vi "png_to_colors.vi"(11 "colors":string(combo)="parula") -> (3 "colors":u32[](array[colorbox]))   [LabVIEW 2019, in "Mandelbrot.lvlib"]
uses:
  Mandelbrot.lvlib
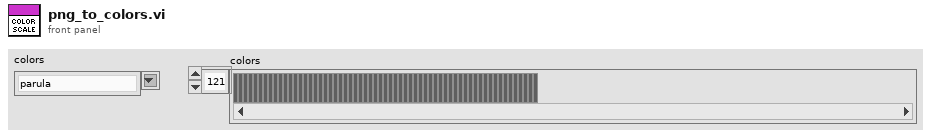
[diagram p1: front panel]
types:
  T1 = typedef "imagedata.ctl" = cluster{"image type":i32, "image depth":i32, "image":u8[], "mask":u8[], "colors":u32[], "Rectangle":cluster{"left":i16, "top":i16, "right":i16, "bottom":i16}}
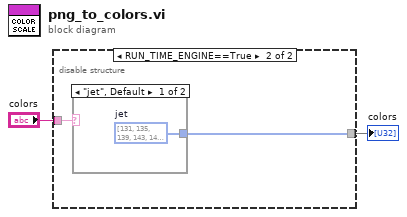
[diagram p0: block diagram]
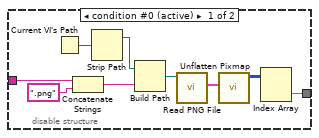
[diagram p2: hidden frame]
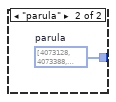
[diagram p3: hidden frame]
diagram:
  n1 = disable-structure shown="RUN_TIME_ENGINE==True" {
    disable-tunnel: [w6 w12] -> w2
    disable-tunnel: "colors" -> [w5 w13]
    frame condition #0 (active) {
      n2 = Current VI's Path() -> (path=w11:path)
      n3 = Concatenate Strings(w5, ".png" ("string")) -> (w3:string)
      n4 = Strip Path(path=w11) -> (stripped path=w10:path)  [unwired: 1 out]
      n5 = Build Path(base path=w10, name or relative path=w3) -> (appended path=w9:path)
      n6 = call <vilib>:"Read PNG File.vi"("path to PNG file"=w9) -> ("image data"=w8:T1)  [unwired: 8 in, 2 out]
      n7 = call <vilib>:"Unflatten Pixmap.vi"("image data"=w8) -> ("24-bit pixmap"=w7:u32[][])  [unwired: 4 in, 6 out]
      n8 = Index Array(array=w7) -> (element=w6:u32[])  [unwired: 2 in]
    }
    frame condition #1 {
      n9 = case shown="\"jet\", Default" w13 {
        tunnel: [w14 w15] -> w12
        frame "jet", Default {
          w14 = u32[] [131, 135, 139, 143, 147, 151, 155, 159, 163, 167, 172, 175, 179, 183, 186, 191, 195, 198, 203, 207, 211, 215, 219, 223, 227, 231, 235, 239, 243, 247, 251, 255, 1279, 2303, 3327, 4607, 5375, 6399, 7423, 8191, 9471, 10495, 11263, 12543, 13567, 14591, 15615, 16639, 17663, 18687, 19711, 20735, 21759, 22783, 23807, 24831, 25855, 26879, 27903, 28927, 30207, 30975, 31999, 33023, 33791, 34815, 35839, 36607, 37887, 38911, 39935, 40959, 41983, 43007, 44031, 45055, 46079, 47103, 48127, 49151, 50175, 51199, 52223, 53247, 54271, 55551, 56319, 57343, 58623, 59391, 60415, 61439, 62207, 63487, 64511, 130814, 327675, 589815, 851955, 1114095, 1376235, 1638375, 1900515, 2162655, 2424795, 2686935, 2949075, 3211215, 3473355, 3735495, 4063170, 4259775, 4521915, 4849590, 5046195, 5308335, 5570475, 5767080, 6094755, 6356895, 6619035, 6881175, 7143315, 7405455, 7667595, 7929735, 8191875, 8454016, 8650620, 8912760, 9174900, 9437040, 9699180, 9961320, 10223460, 10485600, 10747740, 11009880, 11337555, 11534160, 11796300, 12058440, 12255045, 12582720, 12844860, 13041465, 13369140, 13631280, 13893420, 14155560, 14417700, 14679840, 14941980, 15204120, 15466260, 15728400, 15990540, 16252680, 16514820, 16776960, 16775936, 16774912, 16773888, 16772608, 16771840, 16770816, 16769792, 16769024, 16767744, 16766720, 16765952, 16764672, 16763648, 16762624, 16761600, 16760576, 16759552, 16758528, 16757504, 16756480, 16755456, 16754432, 16753408, 16752384, 16751360, 16750336, 16749312, 16748288, 16747008, 16746240, 16745216, 16744448, 16743680, 16742400, 16741376, 16740608, 16739328, 16738304, 16737280, 16736256, 16735232, 16734208, 16733184, 16732160, 16731136, 16730112, 16729088, 16728064, 16727040, 16726016, 16724992, 16723968, 16722944, 16721664, 16720896, 16719872, 16718592, 16717824, 16716800, 16715776, 16715008, 16713728, 16712704, 16646400, 16449536, 16187392, 15925248, 15663104, 15400960, 15138816, 14876672, 14614528, 14352384, 14090240, 13828096, 13565952, 13303808, 13041664, 12713984, 12517376, 12255232, 11927552, 11730944, 11468800, 11206656, 11010048, 10682368, 10420224, 10158080, 9895936, 9633792, 9371648, 9109504, 8847360, 8585216, 8388608]  # jet
        }
        frame "parula" {
          w15 = u32[] [4073128, 4073388, 4139183, 4139442, 4205236, 4205495, 4271290, 4271549, 4337343, 4337602, 4403397, 4403656, 4403914, 4469709, 4469967, 4535762, 4536277, 4536535, 4602329, 4602588, 4602846, 4603360, 4669153, 4669411, 4669925, 4670182, 4670696, 4670953, 4671211, 4737260, 4737517, 4738030, 4738288, 4738801, 4739058, 4739315, 4739828, 4740085, 4740342, 4675319, 4675575, 4676088, 4676345, 4676602, 4677114, 4611835, 4612347, 4612604, 4547324, 4547837, 4482557, 4417533, 4417790, 4352766, 4287486, 4222462, 4157183, 4092159, 3961343, 3896319, 3765503, 3700478, 3569662, 3504637, 3373821, 3308796, 3243516, 3178491, 3113210, 3113722, 3048441, 3048696, 3049208, 3049463, 2984182, 2984693, 2984948, 2985203, 2985714, 2920433, 2920688, 2855407, 2790382, 2725101, 2659820, 2594795, 2595050, 2529769, 2530024, 2464744, 2464999, 2399974, 2400229, 2334949, 2335204, 2269924, 2204643, 2139619, 2074338, 2009057, 1943777, 1944032, 1878751, 1813470, 1748189, 1682908, 1552090, 1486809, 1355992, 1225174, 1094357, 963540, 766930, 570577, 439759, 308942, 178124, 112586, 47305, 47559, 47814, 113348, 179138, 310209, 441535, 638397, 900540, 1097402, 1359544, 1556406, 1753269, 1949875, 2146737, 2343343, 2474670, 2605740, 2737066, 2868136, 2933926, 3064997, 3130787, 3261857, 3327647, 3393437, 3524507, 3590297, 3721366, 3787156, 3918226, 4049552, 4246157, 4377227, 4574089, 4770694, 4967300, 5164161, 5360767, 5557372, 5753978, 5950583, 6212980, 6409586, 6606191, 6868332, 7064937, 7261542, 7523684, 7720034, 7982174, 8244315, 8440921, 8703062, 8964947, 9161553, 9423694, 9685579, 9882184, 10144070, 10340675, 10602560, 10799166, 10995515, 11257657, 11454007, 11716149, 11912499, 12108849, 12305455, 12567341, 12763948, 12960298, 13156649, 13287720, 13549607, 13680423, 13877031, 14073383, 14269992, 14400808, 14597161, 14793770, 14924843, 15121197, 15252270, 15383088, 15514162, 15710773, 15841847, 15972921, 16103995, 16235069, 16366142, 16497470, 16563262, 16694589, 16694844, 16695355, 16695610, 16695865, 16696376, 16696631, 16697141, 16697396, 16697907, 16632626, 16633137, 16633393, 16568368, 16503343, 16503598, 16438574, 16373293, 16373804, 16308523, 16243498, 16244010, 16178729, 16179240, 16113960, 16114471, 16114982, 16115238, 16115749, 16116004, 16116515, 16116770, 16117281, 16183072, 16183583, 16183838, 16249884, 16250139, 16316186, 16316440, 16382230, 16382741]  # parula
        }
      }
    }
  }
  "colors" <- w2
